vi "memmon.vi"() -> ()   [LabVIEW 2011]
panel:
  in  "LIST ALL":bool
  in  "open":bool
  in  "VIs IN MEMORY":i32(listbox)
  in  "LIST NEW":bool
  out "Listed":i32
  out "Total":i32
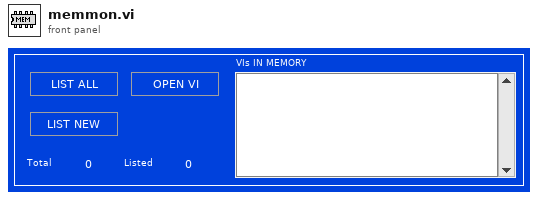
[diagram p1: front panel]
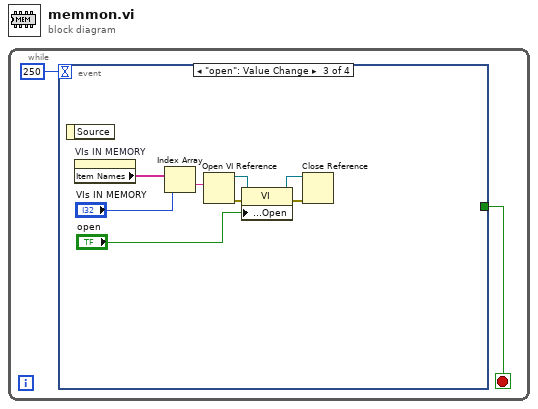
[diagram p0: block diagram]
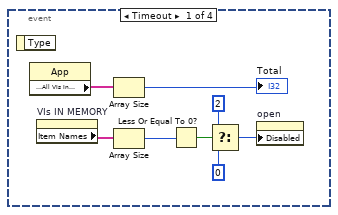
[diagram p2: hidden frame]
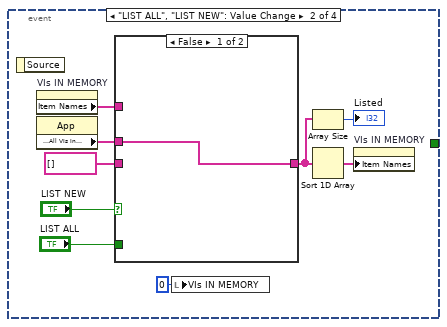
[diagram p3: hidden frame]
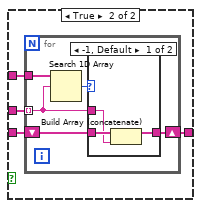
[diagram p4: hidden frame]
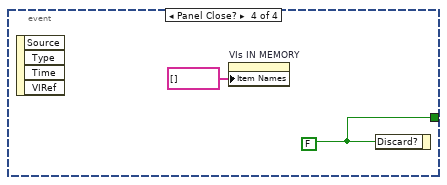
[diagram p6: hidden frame]
diagram:
  n1 = while {
    stop <- w1 stop-if-true
    n2 = event shown="[2] \"open\": Value Change" {
      selector: _ -> [_ _ _ _]
      dyn-events: _ -> [_ _ _ _]
      timeout: 250 -> [_ _ _ _]
      tunnel: [_ _ _ w42] -> w1
      event Timeout {
        n3 = event-data() -> ()  [unwired: 2 out]
        n4 = property class="App"() -> ("Application:All VIs In Memory"=w10:string[])  [unwired: 2 in, 2 out]
        n5 = property on="VIs IN MEMORY" class="LstBox (strict)"() -> ("Item Names"=w5:string[])  [unwired: 2 in, 2 out]
        n6 = Array Size(array=w10) -> (size(s)=→"Total":i32)
        n7 = Array Size(array=w5) -> (size(s)=w4:i32)
        n8 = Less Or Equal To 0?(x=w4) -> (x <= 0?=w3:bool)
        n9 = Select(t=u8 2 ("Disabled"), s=w3, f=u8 0 ("Disabled")) -> (s? t:f=w6:u8)
        n10 = property on="open" class="Bool"("Disabled"=w6) -> ()  [unwired: 2 in, 2 out]
      }
      event "LIST ALL", "LIST NEW": Value Change {
        n11 = event-data() -> ()  [unwired: 2 out]
        n12 = property on="VIs IN MEMORY" class="LstBox (strict)"() -> ("Item Names"=w15:string[])  [unwired: 2 in, 2 out]
        n13 = property class="App"() -> ("Application:All VIs In Memory"=w16:string[])  [unwired: 2 in, 2 out]
        n14 = case shown="False" "LIST NEW" {
          tunnel: [w20 w24] -> w18
          tunnel: w16 -> [w20 w23]
          tunnel: w15 -> [_ w22]
          tunnel: string[] [] ("App.AllVIs") -> [_ w21]
          tunnel: "LIST ALL" -> [_ _]
          frame False {
          }
          frame True {
            n15 = for {
              tunnel: w23 -> [w25] mode=indexing
              tunnel: w22 -> [w29]
              shift-right: [w26] -> w24
              shift-left: w21 -> [w27]
              n16 = Search 1D Array(1D array=w29, element=w25) -> (index of element=w28:i32)  [unwired: 1 out]
              n17 = case shown="-1, Default" w28 {
                tunnel: w27 -> [w32 w33]
                tunnel: [w31 w33] -> w26
                tunnel: w25 -> [w30 _]
                frame -1, Default {
                  n18 = Build Array (concatenate)(w32, w30) -> (w31:string[])
                }
                frame 0.. {
                }
              }
            }
          }
        }
        n19 = local write "VIs IN MEMORY"(0 ("VIs IN MEMORY")) -> ()
        n20 = Array Size(array=w18) -> (size(s)=→"Listed":i32)
        n21 = Sort 1D Array(array=w18) -> (sorted array=w19:string[])
        n22 = property on="VIs IN MEMORY" class="LstBox (strict)"("Item Names"=w19) -> ()  [unwired: 2 in, 2 out]
      }
      event "open": Value Change {
        n23 = event-data() -> ()  [unwired: 2 out]
        n24 = property on="VIs IN MEMORY" class="LstBox (strict)"() -> ("Item Names"=w36:string[])  [unwired: 2 in, 2 out]
        n25 = Index Array(array=w36, index="VIs IN MEMORY") -> (element=w37:string)
        n26 = Open VI Reference(vi path=w37) -> (vi reference=w38:refnum<vi>, error out=w39:errorcluster)  [unwired: 1 in, 4 out]
        n27 = property class="VI"(reference=w38, error in=w39, "Front Panel Window:Open"="open") -> (reference out=w41:refnum<vi>, error out=w40:errorcluster)
        n28 = Close Reference(reference=w41, error in (no error)=w40) -> ()  [unwired: 1 out]
      }
      event Panel Close? {
        w42 = FALSE
        n29 = event-data() -> ()  [unwired: 5 out]
        n30 = property on="VIs IN MEMORY" class="LstBox (strict)"("Item Names"=string[] []) -> ()  [unwired: 2 in, 2 out]
        n31 = event-data("Discard?"=w42) -> ()  [unwired: 1 in, 1 out]
      }
    }
  }
